vi "Load dat File.vi"(8 "error in":errorcluster, 9 "Read only header? (F)":bool, 11 "File path":path) -> (0 "error out":errorcluster, 1 "Data":sgl[][](array[numeric]), 2 "Channels names":string[](array[string]), 3 "Attributes":string[][](array[string]))   [LabVIEW 2016, in "Nanonis Prog Interface.lvlib"]
doc: "<b>Loads a .dat file.</b>\n\nIt returns the header information (attributes), the channels names, and the data of a .dat file.\n\n<B>File path</B>: the full path of the file to load. If empty, a dialog window will open.\n<B>Read only header</B>: if True, the data won't be loaded, only the header information. It is set to False by default.\n\n<B>Attributes</B>: the first column contains the attribute name, and the second column contains the attribute value.\n<B>Channels names</B>: the names of the channels saved in the file.\n<B>Data</B>: loaded data in 2D array format.\n\n- Nanonis Programming Interface -"
uses:
  Nanonis Prog Interface.lvlib
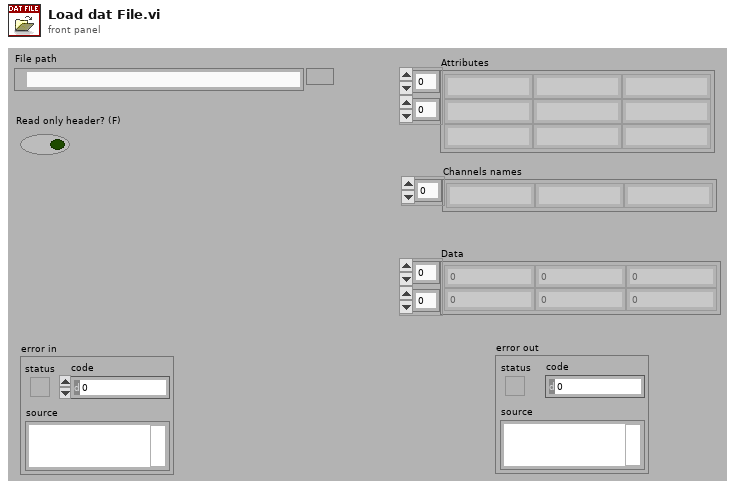
[diagram p1: front panel]
types:
  T1 = enum16{"open", "replace", "create", "open or create", "replace or create", "replace or create with confirmation"}
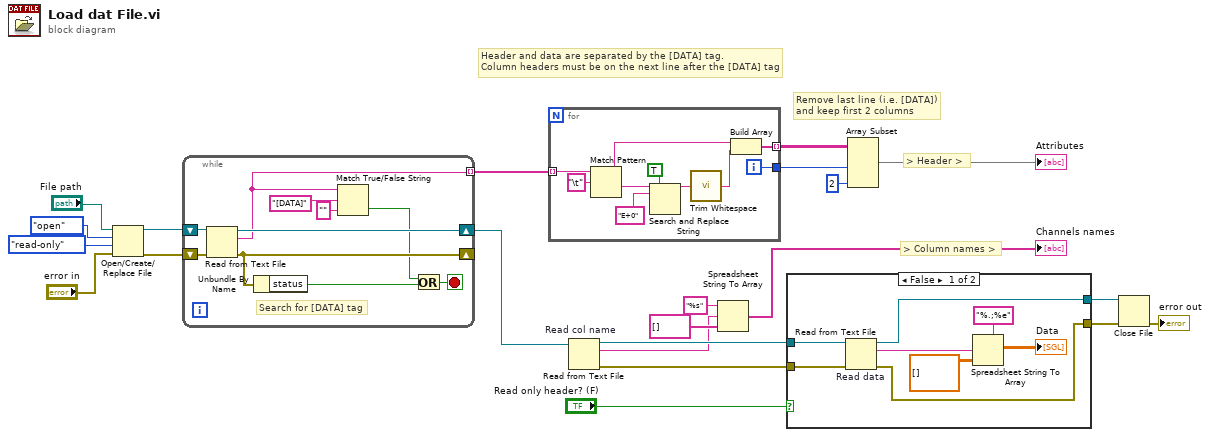
[diagram p0: block diagram]
diagram:
  # "> Column names >"
  # "Remove last line (i.e. [DATA])\nand keep first 2 columns"
  # "> Header >"
  # "Header and data are separated by the [DATA] tag.\nColumn headers must be on the next line after the [DATA] tag"
  n1 = Open/Create/Replace File(file path (use dialog)="File path", error in="error in", operation (0:open)=T1."open", access (0:read/write)=enum16{"read/write", "read-only", "write-only"}."read-only") -> (refnum out=w18:refnum<file>, error out=w12:errorcluster)  [unwired: 2 in, 1 out]
  n2 = while {
    tunnel: [w26] -> w17 mode=indexing
    shift-right: [w29] -> w5
    shift-left: w18 -> [w32]
    shift-right: [w27] -> _
    shift-left: w12 -> [w28]
    stop <- w30 stop-if-true
    # "Search for [DATA] tag"
    n3 = Read from Text File(file (use dialog)=w32, error in=w28) -> (refnum out=w29:refnum<file>, text=w26:string, error out=w27:errorcluster)  [unwired: 2 in, 1 out]
    n4 = Unbundle By Name(w27) -> ("status"=w31:bool)
    n5 = Match True/False String(2:"" ("false string"), 3:"[DATA]" ("x"), 4:w26) -> (0:w23:bool)  [unwired: 1 out]
    n6 = Or(x=w23, y=w31) -> (x .or. y?=w30:bool)
  }
  n7 = for {
    tunnel: [w35] -> w9 mode=indexing
    tunnel: w17 -> [w41] mode=indexing
    tunnel: [w42] -> w10
    i -> [w42]
    n8 = Match Pattern(string=w41, regular expression="\t") -> (before substring=w36:string, after substring=w39:string)  [unwired: 1 in, 2 out]
    n9 = Search and Replace String(replace all?=TRUE ("replace all? (F)"), input string=w39, search string="E+0") -> (result string=w34:string)  [unwired: 5 in, 3 out]
    n10 = call <vilib>:"Trim Whitespace.vi"("string"=w34) -> ("trimmed string"=w33:string)  [unwired: 1 in]
    n11 = Build Array(w36, w33) -> (w35:string[])
  }
  n12 = Read from Text File "Read col name"(file (use dialog)=w5) -> (refnum out=w14:refnum<file>, text=w6:string, error out=w15:errorcluster)  [unwired: 3 in, 1 out]
  n13 = Spreadsheet String To Array(format string="%s", spreadsheet string=w6, array type (2D Dbl)=string[] []) -> (array=→"Channels names":string[])  [unwired: 1 in]
  n14 = case shown="False" "Read only header? (F)" {
    tunnel: w15 -> [w46 w51]
    tunnel: w14 -> [w45 w52]
    tunnel: [w44 w52] -> w13
    tunnel: [w43 w51] -> w4
    frame False {
      n15 = Read from Text File "Read data"(file (use dialog)=w45, error in=w46) -> (refnum out=w44:refnum<file>, text=w47:string, error out=w43:errorcluster)  [unwired: 2 in, 1 out]
      n16 = Spreadsheet String To Array(format string="%.;%e", spreadsheet string=w47, array type (2D Dbl)=sgl[][] []) -> (array=→"Data":sgl[][])  [unwired: 1 in]
    }
    frame True {
    }
  }
  n17 = Array Subset(array=w9, length (row)=w10, length (col)=2 ("dimension size")) -> (→"Attributes":string[][])  [unwired: 2 in]
  n18 = Close File(refnum=w13, error in=w4) -> (error out=→"error out":errorcluster)  [unwired: 1 out]
